vi "APS set sscnet servo monitor src.vi"(8 "error in (no error)":errorcluster caption="错误输入（无错误）", 9 "Mon_Src":i32, 10 "Mon_No":i32, 11 "Axis_ID":i32) -> (0 "error out":errorcluster caption="错误输出", 3 "function return":i32)   [LabVIEW 2011, in "APS168.lvlib"]
doc: "I32 FNTYPE APS_set_sscnet_servo_monitor_src( I32 Axis_ID, I32 Mon_No, I32 Mon_Src );"
uses:
  APS168.lvlib
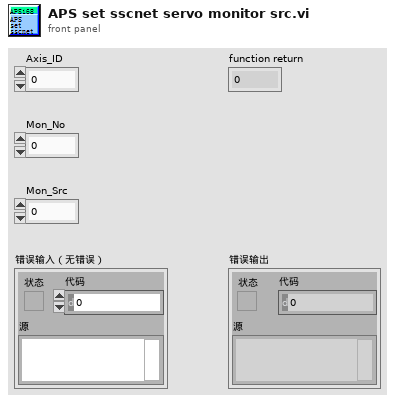
[diagram p1: front panel]
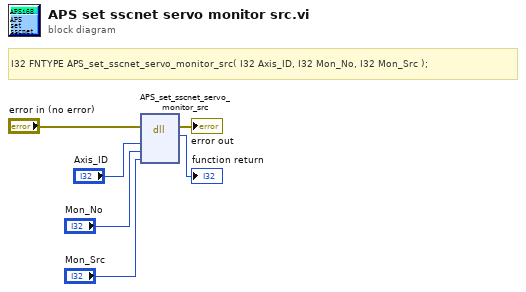
[diagram p0: block diagram]
diagram:
  # "I32 FNTYPE APS_set_sscnet_servo_monitor_src( I32 Axis_ID, I32 Mon_No, I32 Mon_Src );"
  n1 = dll-call lib="PTH1Labs E软件ADLINK 204CAPS_1_7_1_LIB line 连续运动204APS168.*" fn="APS_set_sscnet_servo_monitor_src"(error in="error in (no error)", "Axis_ID"="Axis_ID", "Mon_No"="Mon_No", "Mon_Src"="Mon_Src") -> (error out=→"error out":errorcluster, →"function return":i32)  [unwired: 5 in, 1 out]
